vi "HardWare_Devices Management UI.vi"() -> ()   [LabVIEW 2016]
doc: "搜索系统中网络设备信息\n通过勾选确定需要连接的设备"
uses:
  Ctrls/Wizard_Scan Button.ctl
  Ctrls/Wizard_OK Button.ctl
  Ctrls/Wizard_Cancel Button.ctl
  <vilib>/Utility/error.llb/DialogType.ctl
  Architecture/Queue Management/ARC_Queue Create_Single.vi
  Architecture/Queue Management/ARC_Queue Valid.vi
  Architecture/Queue Management/ARC_Queue Insert Element.vi
  Architecture/Queue Management/ARC_Queue Remove Element.vi
  Architecture/Queue Management/ARC_Queue Destroy_Single.vi
panel:
  in  "Cancel":T1
  in  "OK":T2
  in  "Scan":T3
  out "DevList":i32(listbox) caption="网络设备列表"
  out "Error Report":string
  out "Current State":string
  in  "TempVariable":T4
  in  "Parameter":cluster{"Q-Local":string, "Variant":variant}
  # "/* -------- Notes for All Users -------- */\nRecommand : \n[1].Display Setting Resolution -> 1440x900\n[2].Read Arch Notes First.\n[3].Make A Call When You Are In Trouble.\n\nTeam Members:\nPansino Soft,Pansino SDMA\n\nCopyright@2013 Pansino.Beijing\n\nVersion Number: 2013"
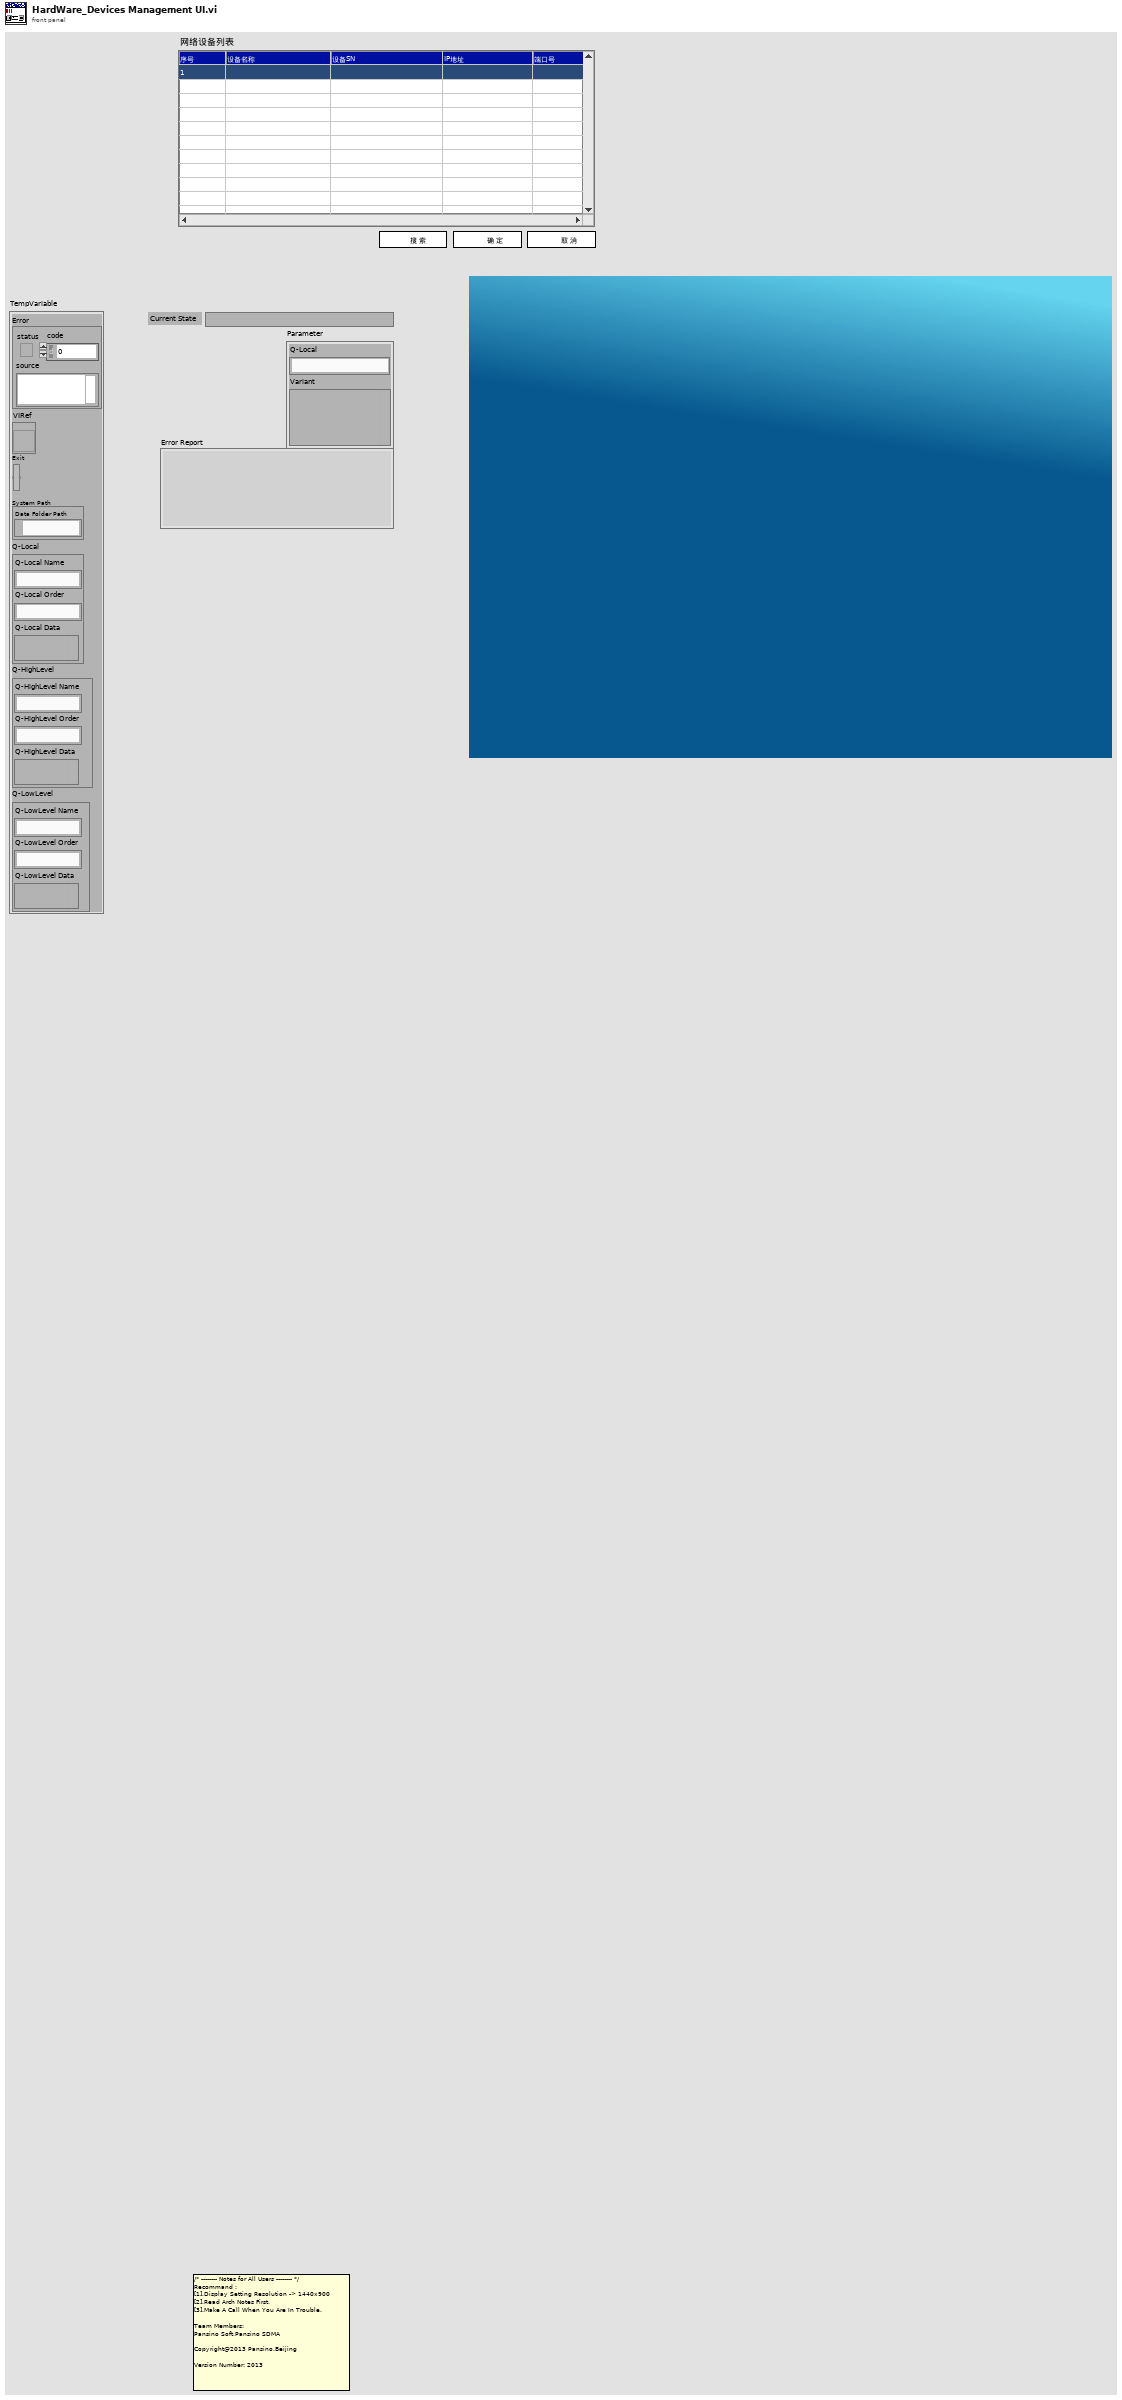
[diagram p1: front panel]
types:
  T1 = typedef "Wizard_Cancel Button.ctl" = bool
  T2 = typedef "Wizard_OK Button.ctl" = bool
  T3 = typedef "Wizard_Scan Button.ctl" = bool
  T4 = cluster{"Error":errorcluster, "VIRef":refnum<vi>, "Exit":bool, "System Path":cluster{"Data Folder Path":path}, "Q-Local":cluster{"Q-Local Name":string, "Q-Local Order":string, "Q-Local Data":variant}, "Q-HighLevel":cluster{"Q-HighLevel Name":string, "Q-HighLevel Order":string, "Q-HighLevel Data":variant}, "Q-LowLevel":cluster{"Q-LowLevel Name":string, "Q-LowLevel Order":string, "Q-LowLevel Data":variant}}
  T5 = typedef "DialogType.ctl" = u16
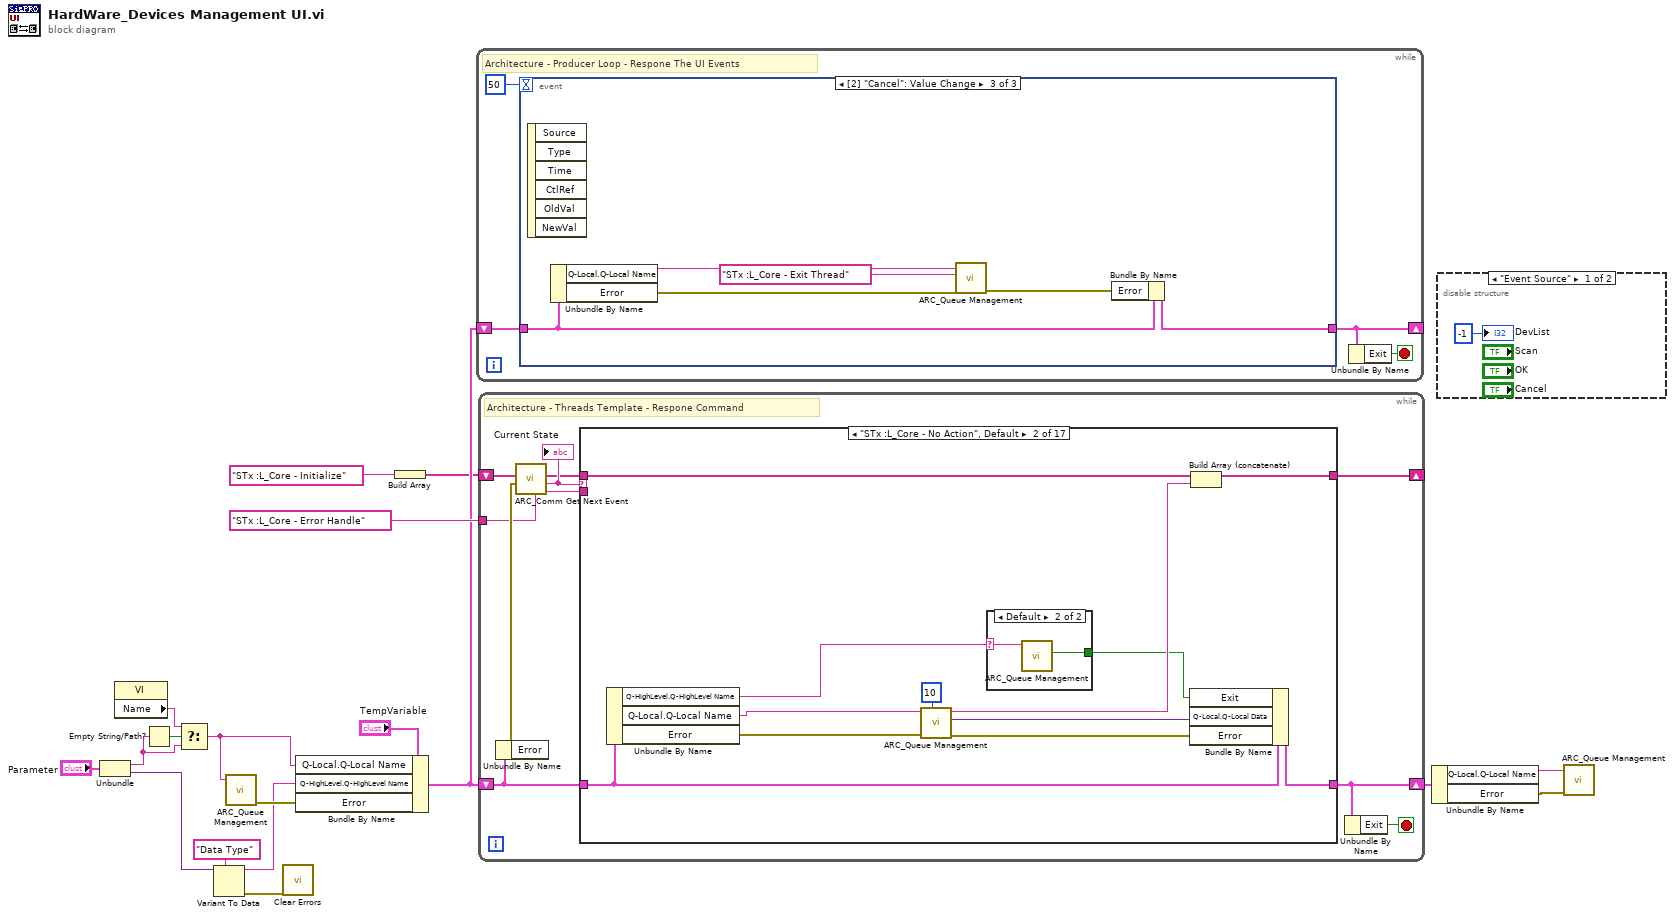
[diagram p0: block diagram]
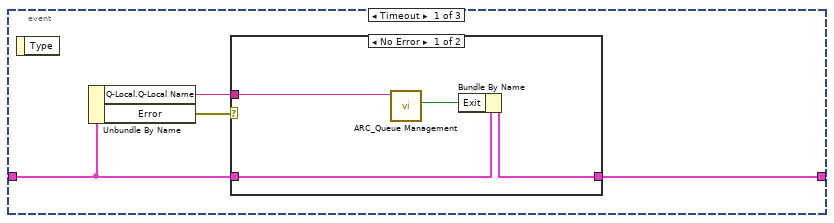
[diagram p2: hidden frame]
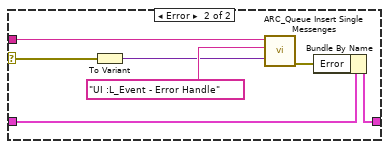
[diagram p3: hidden frame]
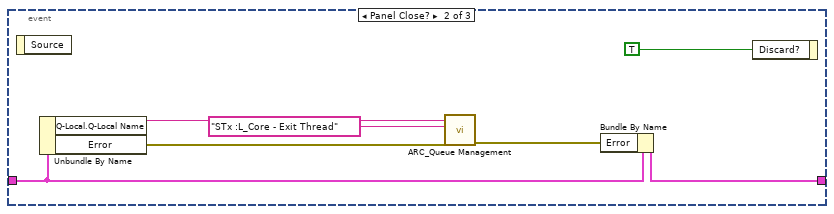
[diagram p4: hidden frame]
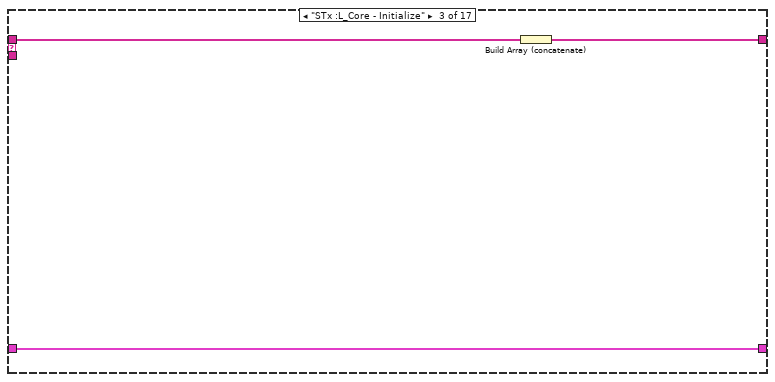
[diagram p8: hidden frame]
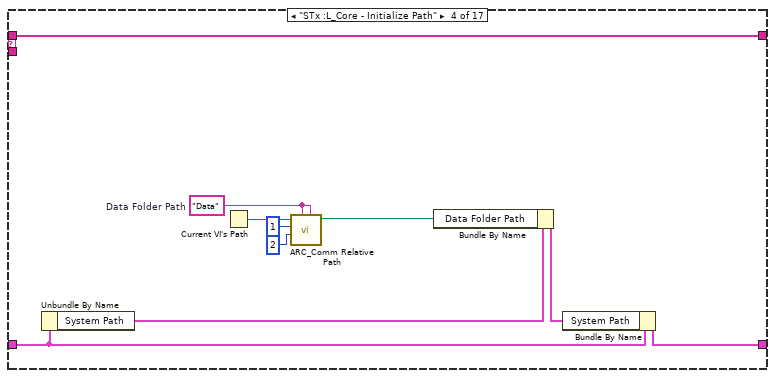
[diagram p9: hidden frame]
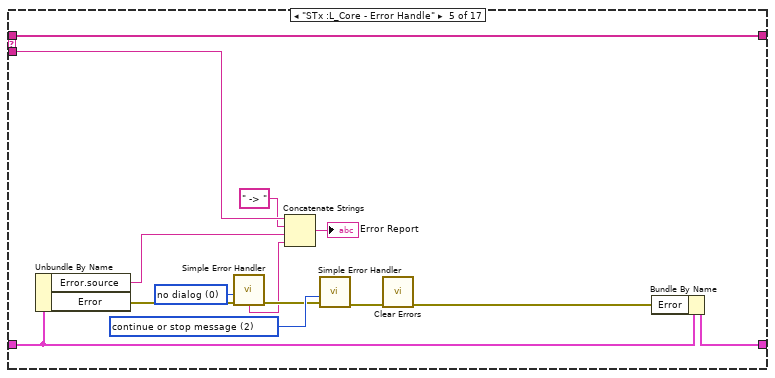
[diagram p10: hidden frame]
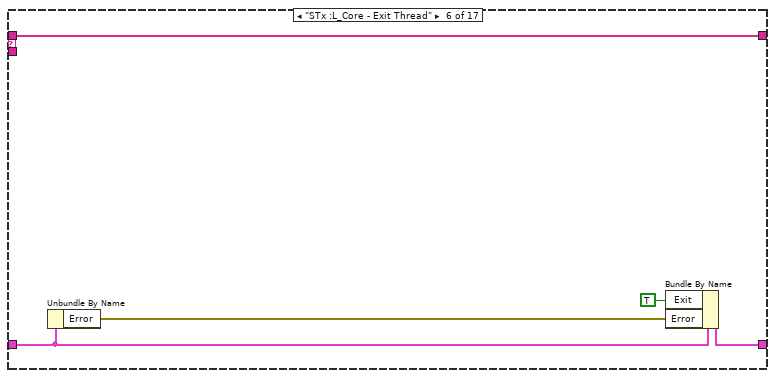
[diagram p11: hidden frame]
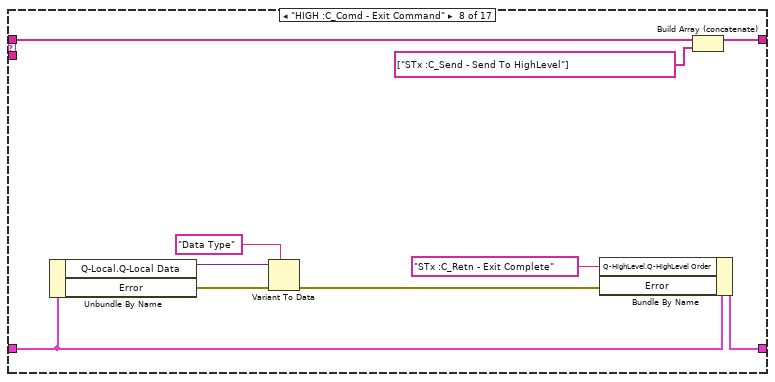
[diagram p13: hidden frame]
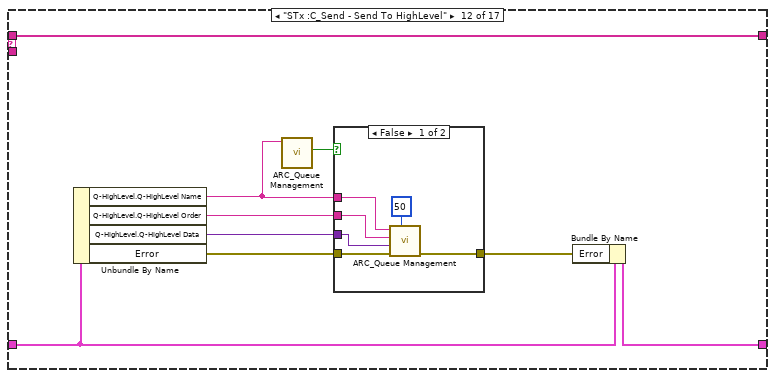
[diagram p17: hidden frame]
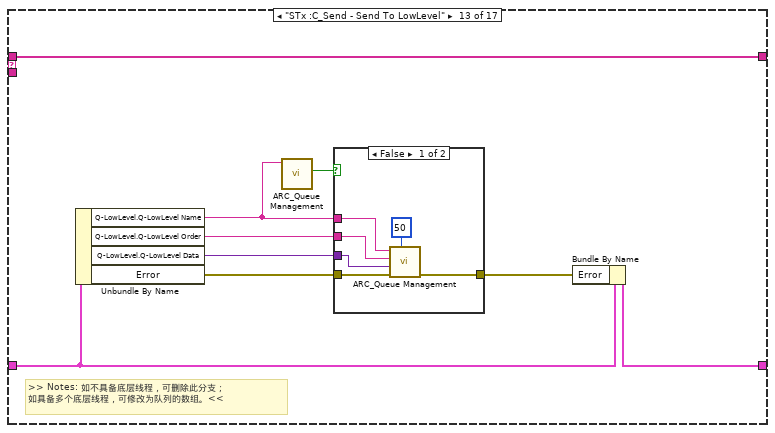
[diagram p19: hidden frame]
diagram:
  n1 = Unbundle("Parameter") -> ("Q-Local"=w3:string, "Variant"=w15:variant)
  n2 = property class="VI"() -> ("Name"=w1:string)  [unwired: 2 in, 2 out]
  n3 = Empty String/Path?(string/path=w3) -> (empty?=w4:bool)
  n4 = Select(t=w1, s=w4, f=w3) -> (s? t:f=w2:string)
  n5 = Variant To Data(type="Data Type" ("Q-Command"), Variant=w15) -> (data=w16:string, error out=w5:errorcluster)  [unwired: 1 in]
  n6 = call-poly "ARC_Queue Management.vi"("Queue Name"=w2) -> ("error out"=w17:errorcluster)  [unwired: 8 in, 2 out]
  n7 = call <vilib>:"Clear Errors.vi"("error in (no error)"=w5) -> ()  [unwired: 5 in, 2 out]
  n8 = Bundle By Name(cluster="TempVariable", "Q-Local.Q-Local Name"=w2, "Q-HighLevel.Q-HighLevel Name"=w16, "Error"=w17) -> (w8:T4)
  n9 = Build Array("STx :L_Core - Initialize") -> (w6:string[])
  n10 = while {
    shift-right: [w20] -> _
    shift-left: w8 -> [w21]
    stop <- w19 stop-if-true
    # "Architecture - Producer Loop - Respone The UI Events"
    n11 = event shown="[2] \"Cancel\": Value Change" {
      selector: _ -> [_ _ _]
      dyn-events: _ -> [_ _ _]
      timeout: 50 -> [_ _ _]
      tunnel: w21 -> [w25 w42 w48]
      tunnel: [w26 w41 w47] -> w20
      event Timeout {
        n12 = event-data() -> ()  [unwired: 1 in, 1 out]
        n13 = Unbundle By Name(w25) -> ("Q-Local.Q-Local Name"=w24:string, "Error"=w23:errorcluster)
        n14 = case shown="No Error" w23 {
          selector: w23 -> [_ w37]
          tunnel: [w30 w35] -> w26
          tunnel: w25 -> [w28 w36]
          tunnel: w24 -> [w27 w34]
          frame No Error {
            n15 = call-poly "ARC_Queue Management.vi"("Queue Name(unamed)"=w27) -> ("Not Exist?"=w29:bool)  [unwired: 8 in, 2 out]
            n16 = Bundle By Name(cluster=w28, "Exit"=w29) -> (w30:T4)
          }
          frame Error {
            n17 = To Variant(anything=w37) -> (Variant=w32:variant)
            n18 = call "ARC_Queue Insert Single Messenges.vi"("Data"=w32, "Order"="UI :L_Event - Error Handle" ("Event"), "Queue Name"=w34) -> ("error out"=w31:errorcluster)  [unwired: 8 in]
            n19 = Bundle By Name(cluster=w36, "Error"=w31) -> (w35:T4)
          }
        }
      }
      event Panel Close? {
        n20 = event-data() -> ()  [unwired: 1 in, 1 out]
        n21 = Unbundle By Name(w42) -> ("Q-Local.Q-Local Name"=w39:string, "Error"=w43:errorcluster)
        n22 = call-poly "ARC_Queue Management.vi"("error in (no error)"=w43, "Event"="STx :L_Core - Exit Thread", "Queue Name(unamed)"=w39) -> ("error out"=w40:errorcluster)  [unwired: 7 in, 1 out]
        n23 = Bundle By Name(cluster=w42, "Error"=w40) -> (w41:T4)
        n24 = event-data("Discard?"=TRUE ("放弃？")) -> ()  [unwired: 1 in, 1 out]
      }
      event Value Change {
        n25 = event-data() -> ()  [unwired: 1 in, 6 out]
        n26 = Unbundle By Name(w48) -> ("Q-Local.Q-Local Name"=w45:string, "Error"=w49:errorcluster)
        n27 = call-poly "ARC_Queue Management.vi"("error in (no error)"=w49, "Event"="STx :L_Core - Exit Thread", "Queue Name(unamed)"=w45) -> ("error out"=w46:errorcluster)  [unwired: 7 in, 1 out]
        n28 = Bundle By Name(cluster=w48, "Error"=w46) -> (w47:T4)
      }
    }
    n29 = Unbundle By Name(w20) -> ("Exit"=w19:bool)
  }
  n30 = while {
    shift-right: [w54] -> w13
    shift-left: w8 -> [w56]
    shift-right: [w57] -> _
    shift-left: w6 -> [w60]
    tunnel: "STx :L_Core - Error Handle" ("Error Handle") -> [w52]
    stop <- w53 stop-if-true
    # "Architecture - Threads Template - Respone Command"
    n31 = Unbundle By Name(w56) -> ("Error"=w55:errorcluster)
    n32 = call "ARC_Comm Get Next Event.vi"("Error Handle"=w52, "error in (no error)"=w55, "event queue in"=w60) -> ("prev event"=w51:string, "next event"=w59:string, "event queue out"=w58:string[])  [unwired: 3 in]
    "Current State" <- w59
    n33 = case shown="\"STx :L_Core - No Action\", Default" w59 {
      tunnel: w56 -> [w61 w74 w78 w87 w101 w105 w109 w117 w121 w123 w125 w132 w148 w159 w164 w171 w177]
      tunnel: w58 -> [w62 w72 w79 w89 w103 w108 w110 w120 w122 w124 w126 w135 w151 w160 w162 w172 w175]
      tunnel: [w62 w71 w77 w89 w103 w108 w110 w118 w122 w124 w126 w135 w151 w160 w161 w172 w174] -> w57
      tunnel: [w61 w73 w78 w88 w102 w106 w109 w119 w121 w123 w125 w131 w147 w159 w163 w170 w176] -> w54
      tunnel: w51 -> [_ _ _ _ w94 _ _ _ _ _ _ _ _ _ _ _ _]
      frame "----------Core Status----------" {
      }
      frame "STx :L_Core - No Action", Default {
        n34 = Unbundle By Name(w74) -> ("Q-HighLevel.Q-HighLevel Name"=w64:string, "Q-Local.Q-Local Name"=w65:string, "Error"=w67:errorcluster)
        n35 = call-poly "ARC_Queue Management.vi"("Time out(-1)_queue out"=10, "error in (no error)"=w67, "Queue Name(unamed)"=w65) -> ("error out"=w69:errorcluster, "Data"=w68:variant, "Event"=w70:string)  [unwired: 5 in, 1 out]
        n36 = case shown="Default" w64 {
          selector: w64 -> [_ w75]
          tunnel: [_ w76] -> w66
          frame "" {
          }
          frame Default {
            n37 = call-poly "ARC_Queue Management.vi"("Queue Name(unamed)"=w75) -> ("Not Exist?"=w76:bool)  [unwired: 8 in, 2 out]
          }
        }
        n38 = Bundle By Name(cluster=w74, "Exit"=w66, "Q-Local.Q-Local Data"=w68, "Error"=w69) -> (w73:T4)
        n39 = Build Array (concatenate)(w72, w70) -> (w71:string[])
      }
      frame "STx :L_Core - Initialize" {
        n40 = Build Array (concatenate)(w79) -> (w77:string[])
      }
      frame "STx :L_Core - Initialize Path" {
        w82 = "Data"  # Data Folder Path
        n41 = Unbundle By Name(w87) -> ("System Path"=w81:cluster{"Data Folder Path":path})
        n42 = Current VI's Path() -> (path=w83:path)
        n43 = call "ARC_Comm Relative Path.vi"("Development Relative Path"=w82, "Run Time relative path"=w82, "Run-Time File Depth"=2, "Development File Depth"=1, "Root Path"=w83) -> ("Relative Path"=w86:path)  [unwired: 5 in, 1 out]
        n44 = Bundle By Name(cluster=w81, "Data Folder Path"=w86) -> (w80:cluster{"Data Folder Path":path})
        n45 = Bundle By Name(cluster=w87, "System Path"=w80) -> (w88:T4)
      }
      frame "STx :L_Core - Error Handle" {
        w95 = T5 0 items=["no dialog", "OK message", "continue or stop message", "OK message + warnings", "continue/stop + warnings"] ("type of dialog (OK msg:1)")
        w98 = T5 2 items=["no dialog", "OK message", "continue or stop message", "OK message + warnings", "continue/stop + warnings"] ("type of dialog (OK msg:1)")
        n46 = Unbundle By Name(w101) -> ("Error.source"=w90:string, "Error"=w97:errorcluster)
        n47 = call <vilib>:"Simple Error Handler.vi"("type of dialog (OK msg:1)"=w95, "error in (no error)"=w97) -> ("error out"=w96:errorcluster, "message"=w92:string)  [unwired: 3 in, 3 out]
        n48 = Concatenate Strings(w94, " -> " ("字符串"), w90, w92) -> (→"Error Report":string)
        n49 = call <vilib>:"Simple Error Handler.vi"("type of dialog (OK msg:1)"=w98, "error in (no error)"=w96) -> ("error out"=w100:errorcluster)  [unwired: 3 in, 4 out]
        n50 = call <vilib>:"Clear Errors.vi"("error in (no error)"=w100) -> ("error out"=w99:errorcluster)  [unwired: 5 in, 1 out]
        n51 = Bundle By Name(cluster=w101, "Error"=w99) -> (w102:T4)
      }
      frame "STx :L_Core - Exit Thread" {
        n52 = Unbundle By Name(w105) -> ("Error"=w107:errorcluster)
        n53 = Bundle By Name(cluster=w105, "Exit"=TRUE, "Error"=w107) -> (w106:T4)
      }
      frame "----------Commond From HIGH----------" {
      }
      frame "HIGH :C_Comd - Exit Command" {
        n54 = Unbundle By Name(w117) -> ("Q-Local.Q-Local Data"=w116:variant, "Error"=w115:errorcluster)
        n55 = Variant To Data(error in=w115, type="Data Type" ("Data Type"), Variant=w116) -> (error out=w113:errorcluster)  [unwired: 1 out]
        n56 = Bundle By Name(cluster=w117, "Q-HighLevel.Q-HighLevel Order"="STx :C_Retn - Exit Complete" ("Data Type"), "Error"=w113) -> (w119:T4)
        n57 = Build Array (concatenate)(w120, string[] ["STx :C_Send - Send To HighLevel"] ("数组")) -> (w118:string[])
      }
      frame "----------Actions----------" {
      }
      frame "----------Operation----------" {
      }
      frame "----------Communication----------" {
      }
      frame "STx :C_Send - Send To HighLevel" {
        n58 = Unbundle By Name(w132) -> ("Q-HighLevel.Q-HighLevel Name"=w134:string, "Q-HighLevel.Q-HighLevel Order"=w129:string, "Q-HighLevel.Q-HighLevel Data"=w128:variant, "Error"=w133:errorcluster)
        n59 = call-poly "ARC_Queue Management.vi"("Queue Name(unamed)"=w134) -> ("Not Exist?"=w130:bool)  [unwired: 8 in, 2 out]
        n60 = case shown="False" w130 {
          tunnel: w133 -> [w141 w142]
          tunnel: w134 -> [w139 _]
          tunnel: w129 -> [w137 _]
          tunnel: w128 -> [w138 _]
          tunnel: [w136 w142] -> w127
          frame False {
            n61 = call-poly "ARC_Queue Management.vi"("Time out(-1)_queue in"=50, "error in (no error)"=w141, "Data"=w138, "Event"=w137, "Queue Name(unamed)"=w139) -> ("error out"=w136:errorcluster)  [unwired: 5 in, 1 out]
          }
          frame True {
          }
        }
        n62 = Bundle By Name(cluster=w132, "Error"=w127) -> (w131:T4)
      }
      frame "STx :C_Send - Send To LowLevel" {
        # ">> Notes: 如不具备底层线程，可删除此分支；\n如具备多个底层线程，可修改为队列的数组。<<"
        n63 = Unbundle By Name(w148) -> ("Q-LowLevel.Q-LowLevel Name"=w150:string, "Q-LowLevel.Q-LowLevel Order"=w145:string, "Q-LowLevel.Q-LowLevel Data"=w144:variant, "Error"=w149:errorcluster)
        n64 = call-poly "ARC_Queue Management.vi"("Queue Name(unamed)"=w150) -> ("Not Exist?"=w146:bool)  [unwired: 8 in, 2 out]
        n65 = case shown="False" w146 {
          tunnel: w149 -> [w157 w158]
          tunnel: w150 -> [w155 _]
          tunnel: w145 -> [w153 _]
          tunnel: w144 -> [w154 _]
          tunnel: [w152 w158] -> w143
          frame False {
            n66 = call-poly "ARC_Queue Management.vi"("Time out(-1)_queue in"=50, "error in (no error)"=w157, "Data"=w154, "Event"=w153, "Queue Name(unamed)"=w155) -> ("error out"=w152:errorcluster)  [unwired: 5 in, 1 out]
          }
          frame True {
          }
        }
        n67 = Bundle By Name(cluster=w148, "Error"=w143) -> (w147:T4)
      }
      frame "----------Respond From LOW----------" {
      }
      frame "LOW :C_Resp - /* ADD NAME */" {
        n68 = Unbundle By Name(w164) -> ("Error"=w165:errorcluster)
        n69 = Build Array (concatenate)(w162) -> (w161:string[])
        n70 = Bundle By Name(cluster=w164, "Error"=w165) -> (w163:T4)
      }
      frame "LOW :C_Resp - /*Respond The Request*/" {
        n71 = Unbundle By Name(w171) -> ("Q-Local.Q-Local Data"=w168:variant, "Error"=w169:errorcluster)
        n72 = Variant To Data(error in=w169, type="Data Type" ("Data Type"), Variant=w168) -> (error out=w167:errorcluster)  [unwired: 1 out]
        n73 = Bundle By Name(cluster=w171, "Error"=w167) -> (w170:T4)
      }
      frame "LOW :C_Resp - Exit Complete" {
        # ">> Notes: 此处接收下层的返回指令；: 前代表下层的VI功能名，如ACTS等<<"
        n74 = Unbundle By Name(w177) -> ("Error"=w178:errorcluster)
        n75 = Build Array (concatenate)(w175, string[] ["STx :L_Core - Exit Thread"] ("数组")) -> (w174:string[])
        n76 = Bundle By Name(cluster=w177, "Error"=w178) -> (w176:T4)
      }
    }
    n77 = Unbundle By Name(w54) -> ("Exit"=w53:bool)
  }
  n78 = Unbundle By Name(w13) -> ("Q-Local.Q-Local Name"=w11:string, "Error"=w12:errorcluster)
  n79 = disable-structure shown="\"Event Source\"" {
    frame condition #0 (active) {
      "DevList" <- -1 ("DevList")
    }
    frame condition #1 {
    }
  }
  n80 = call-poly "ARC_Queue Management.vi"("error in (no error)"=w12, "Queue Name(unamed)"=w11) -> ()  [unwired: 7 in, 3 out]
